vi "LS370_read_only_Open_Queue.vi"(8 "error in (no error)":errorcluster) -> (0 "error out":errorcluster, 2 "queue out":refnum<queue>)   [LabVIEW 2019]
uses:
  LS370/LS370_read_only_control.ctl
  Global/Global Variables/Queues_global.vi
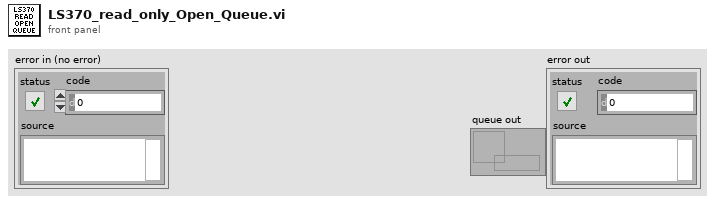
[diagram p1: front panel]
types:
  T1 = typedef "LS370_read_only_control.ctl" = cluster{"Update Lakeshores":bool}
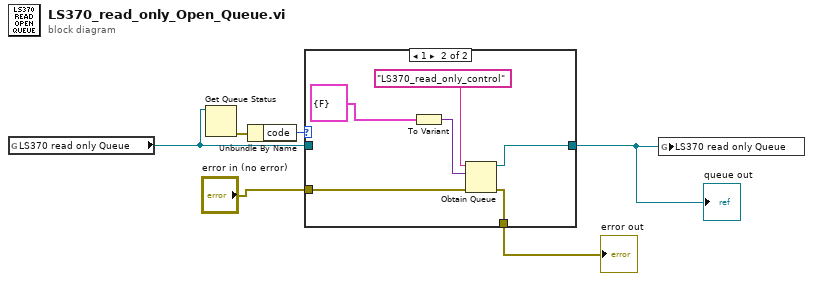
[diagram p0: block diagram]
diagram:
  n1 = global read "Queues_global.vi" "LS370 read only Queue"() -> (w4:refnum<queue>)
  n2 = Get Queue Status(queue=w4) -> (error out=w6:errorcluster)  [unwired: 2 in, 7 out]
  n3 = Unbundle By Name(w6) -> ("code"=w5:i32)
  n4 = case shown="1" w5 {
    tunnel: [w8 w12] -> w3
    tunnel: w4 -> [w8 _]
    tunnel: "error in (no error)" -> [w7 w10]
    tunnel: [w7 w9] -> w1
    frame 0, Default {
    }
    frame 1 {
      n5 = To Variant(anything=T1 {"Update Lakeshores"=FALSE} ("Lakeshore 370 read only Control")) -> (Variant=w13:variant)
      n6 = Obtain Queue(name (unnamed)="LS370_read_only_control", element data type=w13, error in (no error)=w10) -> (queue out=w12:refnum<queue>, error out=w9:errorcluster)  [unwired: 2 in, 1 out]
    }
  }
  "queue out" <- w3
  "error out" <- w1
  n7 = global write "Queues_global.vi" "LS370 read only Queue"(w3) -> ()
